vi "PicoScopeospaExampleRapidBlockBulkOverlapped.vi"() -> ()   [LabVIEW 2010]
uses:
  shared/PicoBuffers.ctl
  <vilib>/Waveform/DWDTOps.llb/DWDT Analog to Digital.vi
  PicoScopepsospaLib/PicoScopeospaDigitalChannelSettings.ctl
  PicoScopepsospaLib/PicoScopeospaAnalogChannelSettings.ctl
  shared/Buffer and Transfer Settings.ctl
  shared/Acquisition Settings.ctl
  shared/Segment Range.ctl
panel:
  in  "timeIntervalRequested":dbl=2e-10 format="%#6_6p"
  in  "Write to file":bool
  in  "Channels":T1={"Channel A Settings "={"Enabled"=TRUE, "Coupling"=1, "Range"=8, "Analogue Offset"=0.0, "BandWidth"=0, "PROBE_RANGE_INFO"=0}, "Channel B Settings "={"Enabled"=FALSE, "Coupling"=1, "Range"=8, "Analogue Offset"=0.0, "BandWidth"=0, "PROBE_RANGE_INFO"=0}, "Channel C Settings "={"Enabled"=FALSE, "Coupling"=1, "Range"=8, "Analogue Offset"=0.0, "BandWidth"=0, "PROBE_RANGE_INFO"=0}, "Channel D Settings "={"Enabled"=FALSE, "Coupling"=1, "Range"=8, "Analogue Offset"=0.0, "BandWidth"=0, "PROBE_RANGE_INFO"=0}, "Channel E Settings "={"Enabled"=FALSE, "Coupling"=50, "Range"=5, "Analogue Offset"=0.0, "BandWidth"=0, "PROBE_RANGE_INFO"=0}, "Channel F Settings "={"Enabled"=FALSE, "Coupling"=50, "Range"=5, "Analogue Offset"=0.0, "BandWidth"=0, "PROBE_RANGE_INFO"=0}, "Channel G Settings "={"Enabled"=FALSE, "Coupling"=50, "Range"=5, "Analogue Offset"=0.0, "BandWidth"=0, "PROBE_RANGE_INFO"=0}, "Channel H Settings "={"Enabled"=FALSE, "Coupling"=50, "Range"=5, "Analogue Offset"=0.0, "BandWidth"=0, "PROBE_RANGE_INFO"=0}} {"Channel H Settings"."PROBE_RANGE_INFO" items=["PROBE_NONE_NV"=0, "X1_PROBE_NV"=1, "X10_PROBE_NV"=10]; "Channel H Settings"."BandWidth" items=["Full"=0, "100kHz"=100000, "20kHz"=200000, "1MHz"=1000000, "20MHz"=20000000, "25MHz"=25000000, "50MHz"=50000000, "200MHz"=200000000, "250MHz"=250000000, "500MHz"=500000000]; "Channel H Settings"."Range" items=["10mV"=0, "20mV"=1, "50mV"=2, "100mV"=3, "200mV"=4, "500mV"=5, "1V"=6, "2V"=7, "5V"=8, "10V"=9, "20V"=10, "50V"=11, "100V"=12, "200V"=13, "x10_Probe_100mV"=32, "x10_Probe_200mV"=33, "x10_Probe_500mV"=34, "x10_Probe_1V"=35, "x10_Probe_2V"=36, "x10_Probe_5V"=37, "x10_Probe_10V"=38, "x10_Probe_20V"=39, "x10_Probe_50V"=40, "x10_Probe_100V"=41, "x10_Probe_200V"=42, "x10_Probe_500V"=43, "CURRENT_CLAMP_60A_2A"=10500, "CURRENT_CLAMP_60A_5A"=10501, "CURRENT_CLAMP_60A_10A"=10502, "CURRENT_CLAMP_60A_20A"=10503, "CURRENT_CLAMP_60A_50A"=10504, "CURRENT_CLAMP_60A_60A"=10505, "CURRENT_CLAMP_60A_V2_0_5A"=10600, "CURRENT_CLAMP_60A_V2_1A"=10601, "CURRENT_CLAMP_60A_V2_2A"=10602, "CURRENT_CLAMP_60A_V2_5A"=10603, "CURRENT_CLAMP_60A_V2_10A"=10604, "CURRENT_CLAMP_60A_V2_20A"=10605, "CURRENT_CLAMP_60A_V2_50A"=10606, "CURRENT_CLAMP_60A_V2_60A"=10607, "RESISTANCE_LEAD_NEG5_TO_20OHM"=7000, "RESISTANCE_LEAD_NEG50_TO_200OHM"=7001, "RESISTANCE_LEAD_NEG500_TO_2KOHM"=7002, "RESISTANCE_LEAD_NEG5K_TO_20KOHM"=7003, "RESISTANCE_LEAD_NEG50K_TO_LEAD_200KOHM"=7004, "RESISTANCE_LEAD_NEG500K_TO_LEAD_2MOHM"=7005, "RESISTANCE_LEAD_DIODE_TEST"=7006, "HT_NEG3_TO_5KV"=8950, "HT_NEG3_TO_10KV"=8951, "HT_NEG5_TO_20KV"=8952, "HT_NEG5_TO_50KV"=8953, "HT_NEG5_TO_100KV"=8954, "HT_NEG3_TO_5KV_INVERTED"=8955, "HT_NEG3_TO_10KV_INVERTED"=8956, "HT_NEG5_TO_20KV_INVERTED"=8957, "HT_NEG5_TO_50KV_INVERTED"=8958, "HT_NEG5_TO_100KV_INVERTED"=8959, "TEMPERATURE_NEG50_TO_150DEGC"=9000, "PRESSURE_SENSOR_-100k-150k_PASCALS"=9100, "PRESSURE_SENSOR_-100k_TO_400k_PASCALS"=9101, "PRESSURE_SENSOR_-200k_TO_800k_PASCALS"=9102, "PRESSURE_SENSOR_-400k_TO_1600k_PASCALS"=9103, "PRESSURE_SENSOR_-400k_TO_3400k_PASCALS"=9104, "PRESSURE_SENSOR_-150k_TO_1350k_PASCALS"=9105]; "Channel H Settings"."Coupling" items=["AC"=0, "DC 1M Ohm"=1, "DC 50 Ohm"=50]; "Channel G Settings"."PROBE_RANGE_INFO" items=["PROBE_NONE_NV"=0, "X1_PROBE_NV"=1, "X10_PROBE_NV"=10]; "Channel G Settings"."BandWidth" items=["Full"=0, "100kHz"=100000, "20kHz"=200000, "1MHz"=1000000, "20MHz"=20000000, "25MHz"=25000000, "50MHz"=50000000, "200MHz"=200000000, "250MHz"=250000000, "500MHz"=500000000]; "Channel G Settings"."Range" items=["10mV"=0, "20mV"=1, "50mV"=2, "100mV"=3, "200mV"=4, "500mV"=5, "1V"=6, "2V"=7, "5V"=8, "10V"=9, "20V"=10, "50V"=11, "100V"=12, "200V"=13, "x10_Probe_100mV"=32, "x10_Probe_200mV"=33, "x10_Probe_500mV"=34, "x10_Probe_1V"=35, "x10_Probe_2V"=36, "x10_Probe_5V"=37, "x10_Probe_10V"=38, "x10_Probe_20V"=39, "x10_Probe_50V"=40, "x10_Probe_100V"=41, "x10_Probe_200V"=42, "x10_Probe_500V"=43, "CURRENT_CLAMP_60A_2A"=10500, "CURRENT_CLAMP_60A_5A"=10501, "CURRENT_CLAMP_60A_10A"=10502, "CURRENT_CLAMP_60A_20A"=10503, "CURRENT_CLAMP_60A_50A"=10504, "CURRENT_CLAMP_60A_60A"=10505, "CURRENT_CLAMP_60A_V2_0_5A"=10600, "CURRENT_CLAMP_60A_V2_1A"=10601, "CURRENT_CLAMP_60A_V2_2A"=10602, "CURRENT_CLAMP_60A_V2_5A"=10603, "CURRENT_CLAMP_60A_V2_10A"=10604, "CURRENT_CLAMP_60A_V2_20A"=10605, "CURRENT_CLAMP_60A_V2_50A"=10606, "CURRENT_CLAMP_60A_V2_60A"=10607, "RESISTANCE_LEAD_NEG5_TO_20OHM"=7000, "RESISTANCE_LEAD_NEG50_TO_200OHM"=7001, "RESISTANCE_LEAD_NEG500_TO_2KOHM"=7002, "RESISTANCE_LEAD_NEG5K_TO_20KOHM"=7003, "RESISTANCE_LEAD_NEG50K_TO_LEAD_200KOHM"=7004, "RESISTANCE_LEAD_NEG500K_TO_LEAD_2MOHM"=7005, "RESISTANCE_LEAD_DIODE_TEST"=7006, "HT_NEG3_TO_5KV"=8950, "HT_NEG3_TO_10KV"=8951, "HT_NEG5_TO_20KV"=8952, "HT_NEG5_TO_50KV"=8953, "HT_NEG5_TO_100KV"=8954, "HT_NEG3_TO_5KV_INVERTED"=8955, "HT_NEG3_TO_10KV_INVERTED"=8956, "HT_NEG5_TO_20KV_INVERTED"=8957, "HT_NEG5_TO_50KV_INVERTED"=8958, "HT_NEG5_TO_100KV_INVERTED"=8959, "TEMPERATURE_NEG50_TO_150DEGC"=9000, "PRESSURE_SENSOR_-100k-150k_PASCALS"=9100, "PRESSURE_SENSOR_-100k_TO_400k_PASCALS"=9101, "PRESSURE_SENSOR_-200k_TO_800k_PASCALS"=9102, "PRESSURE_SENSOR_-400k_TO_1600k_PASCALS"=9103, "PRESSURE_SENSOR_-400k_TO_3400k_PASCALS"=9104, "PRESSURE_SENSOR_-150k_TO_1350k_PASCALS"=9105]; "Channel G Settings"."Coupling" items=["AC"=0, "DC 1M Ohm"=1, "DC 50 Ohm"=50]; "Channel F Settings"."PROBE_RANGE_INFO" items=["PROBE_NONE_NV"=0, "X1_PROBE_NV"=1, "X10_PROBE_NV"=10]; "Channel F Settings"."BandWidth" items=["Full"=0, "100kHz"=100000, "20kHz"=200000, "1MHz"=1000000, "20MHz"=20000000, "25MHz"=25000000, "50MHz"=50000000, "200MHz"=200000000, "250MHz"=250000000, "500MHz"=500000000]; "Channel F Settings"."Range" items=["10mV"=0, "20mV"=1, "50mV"=2, "100mV"=3, "200mV"=4, "500mV"=5, "1V"=6, "2V"=7, "5V"=8, "10V"=9, "20V"=10, "50V"=11, "100V"=12, "200V"=13, "x10_Probe_100mV"=32, "x10_Probe_200mV"=33, "x10_Probe_500mV"=34, "x10_Probe_1V"=35, "x10_Probe_2V"=36, "x10_Probe_5V"=37, "x10_Probe_10V"=38, "x10_Probe_20V"=39, "x10_Probe_50V"=40, "x10_Probe_100V"=41, "x10_Probe_200V"=42, "x10_Probe_500V"=43, "CURRENT_CLAMP_60A_2A"=10500, "CURRENT_CLAMP_60A_5A"=10501, "CURRENT_CLAMP_60A_10A"=10502, "CURRENT_CLAMP_60A_20A"=10503, "CURRENT_CLAMP_60A_50A"=10504, "CURRENT_CLAMP_60A_60A"=10505, "CURRENT_CLAMP_60A_V2_0_5A"=10600, "CURRENT_CLAMP_60A_V2_1A"=10601, "CURRENT_CLAMP_60A_V2_2A"=10602, "CURRENT_CLAMP_60A_V2_5A"=10603, "CURRENT_CLAMP_60A_V2_10A"=10604, "CURRENT_CLAMP_60A_V2_20A"=10605, "CURRENT_CLAMP_60A_V2_50A"=10606, "CURRENT_CLAMP_60A_V2_60A"=10607, "RESISTANCE_LEAD_NEG5_TO_20OHM"=7000, "RESISTANCE_LEAD_NEG50_TO_200OHM"=7001, "RESISTANCE_LEAD_NEG500_TO_2KOHM"=7002, "RESISTANCE_LEAD_NEG5K_TO_20KOHM"=7003, "RESISTANCE_LEAD_NEG50K_TO_LEAD_200KOHM"=7004, "RESISTANCE_LEAD_NEG500K_TO_LEAD_2MOHM"=7005, "RESISTANCE_LEAD_DIODE_TEST"=7006, "HT_NEG3_TO_5KV"=8950, "HT_NEG3_TO_10KV"=8951, "HT_NEG5_TO_20KV"=8952, "HT_NEG5_TO_50KV"=8953, "HT_NEG5_TO_100KV"=8954, "HT_NEG3_TO_5KV_INVERTED"=8955, "HT_NEG3_TO_10KV_INVERTED"=8956, "HT_NEG5_TO_20KV_INVERTED"=8957, "HT_NEG5_TO_50KV_INVERTED"=8958, "HT_NEG5_TO_100KV_INVERTED"=8959, "TEMPERATURE_NEG50_TO_150DEGC"=9000, "PRESSURE_SENSOR_-100k-150k_PASCALS"=9100, "PRESSURE_SENSOR_-100k_TO_400k_PASCALS"=9101, "PRESSURE_SENSOR_-200k_TO_800k_PASCALS"=9102, "PRESSURE_SENSOR_-400k_TO_1600k_PASCALS"=9103, "PRESSURE_SENSOR_-400k_TO_3400k_PASCALS"=9104, "PRESSURE_SENSOR_-150k_TO_1350k_PASCALS"=9105]; "Channel F Settings"."Coupling" items=["AC"=0, "DC 1M Ohm"=1, "DC 50 Ohm"=50]; "Channel E Settings"."PROBE_RANGE_INFO" items=["PROBE_NONE_NV"=0, "X1_PROBE_NV"=1, "X10_PROBE_NV"=10]; "Channel E Settings"."BandWidth" items=["Full"=0, "100kHz"=100000, "20kHz"=200000, "1MHz"=1000000, "20MHz"=20000000, "25MHz"=25000000, "50MHz"=50000000, "200MHz"=200000000, "250MHz"=250000000, "500MHz"=500000000]; "Channel E Settings"."Range" items=["10mV"=0, "20mV"=1, "50mV"=2, "100mV"=3, "200mV"=4, "500mV"=5, "1V"=6, "2V"=7, "5V"=8, "10V"=9, "20V"=10, "50V"=11, "100V"=12, "200V"=13, "x10_Probe_100mV"=32, "x10_Probe_200mV"=33, "x10_Probe_500mV"=34, "x10_Probe_1V"=35, "x10_Probe_2V"=36, "x10_Probe_5V"=37, "x10_Probe_10V"=38, "x10_Probe_20V"=39, "x10_Probe_50V"=40, "x10_Probe_100V"=41, "x10_Probe_200V"=42, "x10_Probe_500V"=43, "CURRENT_CLAMP_60A_2A"=10500, "CURRENT_CLAMP_60A_5A"=10501, "CURRENT_CLAMP_60A_10A"=10502, "CURRENT_CLAMP_60A_20A"=10503, "CURRENT_CLAMP_60A_50A"=10504, "CURRENT_CLAMP_60A_60A"=10505, "CURRENT_CLAMP_60A_V2_0_5A"=10600, "CURRENT_CLAMP_60A_V2_1A"=10601, "CURRENT_CLAMP_60A_V2_2A"=10602, "CURRENT_CLAMP_60A_V2_5A"=10603, "CURRENT_CLAMP_60A_V2_10A"=10604, "CURRENT_CLAMP_60A_V2_20A"=10605, "CURRENT_CLAMP_60A_V2_50A"=10606, "CURRENT_CLAMP_60A_V2_60A"=10607, "RESISTANCE_LEAD_NEG5_TO_20OHM"=7000, "RESISTANCE_LEAD_NEG50_TO_200OHM"=7001, "RESISTANCE_LEAD_NEG500_TO_2KOHM"=7002, "RESISTANCE_LEAD_NEG5K_TO_20KOHM"=7003, "RESISTANCE_LEAD_NEG50K_TO_LEAD_200KOHM"=7004, "RESISTANCE_LEAD_NEG500K_TO_LEAD_2MOHM"=7005, "RESISTANCE_LEAD_DIODE_TEST"=7006, "HT_NEG3_TO_5KV"=8950, "HT_NEG3_TO_10KV"=8951, "HT_NEG5_TO_20KV"=8952, "HT_NEG5_TO_50KV"=8953, "HT_NEG5_TO_100KV"=8954, "HT_NEG3_TO_5KV_INVERTED"=8955, "HT_NEG3_TO_10KV_INVERTED"=8956, "HT_NEG5_TO_20KV_INVERTED"=8957, "HT_NEG5_TO_50KV_INVERTED"=8958, "HT_NEG5_TO_100KV_INVERTED"=8959, "TEMPERATURE_NEG50_TO_150DEGC"=9000, "PRESSURE_SENSOR_-100k-150k_PASCALS"=9100, "PRESSURE_SENSOR_-100k_TO_400k_PASCALS"=9101, "PRESSURE_SENSOR_-200k_TO_800k_PASCALS"=9102, "PRESSURE_SENSOR_-400k_TO_1600k_PASCALS"=9103, "PRESSURE_SENSOR_-400k_TO_3400k_PASCALS"=9104, "PRESSURE_SENSOR_-150k_TO_1350k_PASCALS"=9105]; "Channel E Settings"."Coupling" items=["AC"=0, "DC 1M Ohm"=1, "DC 50 Ohm"=50]; "Channel D Settings"."BandWidth" items=["Full"=0, "100kHz"=100000, "20kHz"=200000, "1MHz"=1000000, "20MHz"=20000000, "25MHz"=25000000, "50MHz"=50000000, "100MHz"=100000000, "200MHz"=200000000, "250MHz"=250000000, "350MHz"=350000000, "500MHz"=500000000]; "Channel D Settings"."PROBE_RANGE_INFO" items=["PROBE_NONE_NV"=0, "X1_PROBE_NV"=1, "X10_PROBE_NV"=10]; "Channel D Settings"."Range" items=["10mV", "20mV", "50mV", "100mV", "200mV", "500mV", "1V", "2V", "5V", "10V", "20V", "50V", "100V", "200V"]; "Channel D Settings"."Coupling" items=["AC"=0, "DC 1M Ohm"=1, "DC 50 Ohm"=50]; "Channel C Settings"."BandWidth" items=["Full"=0, "100kHz"=100000, "20kHz"=200000, "1MHz"=1000000, "20MHz"=20000000, "25MHz"=25000000, "50MHz"=50000000, "100MHz"=100000000, "200MHz"=200000000, "250MHz"=250000000, "350MHz"=350000000, "500MHz"=500000000]; "Channel C Settings"."PROBE_RANGE_INFO" items=["PROBE_NONE_NV"=0, "X1_PROBE_NV"=1, "X10_PROBE_NV"=10]; "Channel C Settings"."Range" items=["10mV", "20mV", "50mV", "100mV", "200mV", "500mV", "1V", "2V", "5V", "10V", "20V", "50V", "100V", "200V"]; "Channel C Settings"."Coupling" items=["AC"=0, "DC 1M Ohm"=1, "DC 50 Ohm"=50]; "Channel B Settings"."BandWidth" items=["Full"=0, "100kHz"=100000, "20kHz"=200000, "1MHz"=1000000, "20MHz"=20000000, "25MHz"=25000000, "50MHz"=50000000, "100MHz"=100000000, "200MHz"=200000000, "250MHz"=250000000, "350MHz"=350000000, "500MHz"=500000000]; "Channel B Settings"."PROBE_RANGE_INFO" items=["PROBE_NONE_NV"=0, "X1_PROBE_NV"=1, "X10_PROBE_NV"=10]; "Channel B Settings"."Range" items=["10mV", "20mV", "50mV", "100mV", "200mV", "500mV", "1V", "2V", "5V", "10V", "20V", "50V", "100V", "200V"]; "Channel B Settings"."Coupling" items=["AC"=0, "DC 1M Ohm"=1, "DC 50 Ohm"=50]; "Channel A Settings"."PROBE_RANGE_INFO" items=["PROBE_NONE_NV"=0, "X1_PROBE_NV"=1, "X10_PROBE_NV"=10]; "Channel A Settings"."Range" items=["10mV", "20mV", "50mV", "100mV", "200mV", "500mV", "1V", "2V", "5V", "10V", "20V", "50V", "100V", "200V"]; "Channel A Settings"."BandWidth" items=["Full"=0, "100kHz"=100000, "20kHz"=200000, "1MHz"=1000000, "20MHz"=20000000, "25MHz"=25000000, "50MHz"=50000000, "100MHz"=100000000, "200MHz"=200000000, "250MHz"=250000000, "350MHz"=350000000, "500MHz"=500000000]; "Channel A Settings"."Coupling" items=["AC"=0, "DC 1M Ohm"=1, "DC 50 Ohm"=50]}
  out "overflow":i16[](array[numeric])=[1023] format="%010d"
  out "Trigger Offsets":cluster{"Samples":u64, "Time (seconds)":dbl}[](array[cluster]) {"Time (seconds)" format="%#_5p"}
  in  "Stop Display":bool
  out "Capture Complete":bool
  in  "Run":bool
  in  "Display Buffer Index":i32
  in  "Segment Range":T2={"fromSegmentIndex"=0, "toSegmentIndex"=9} {"toSegmentIndex" format="%.4p"; "fromSegmentIndex" format="%.4p"}
  in  "nSegments":u64=10 format="%.4p"
  out "error out":errorcluster
  in  "Data file":path=path "PicoScopeospaExampleRapidBlock ChA Data"
  in  "Digital Channels":T3={"Port 0 Settings "={"Enabled"=FALSE, "Threshold Level (Volts)"=3.0}, "Port 1 Settings"={"Enabled"=FALSE, "Threshold Level (Volts)"=3.0}} {"Port 1 Settings"."Threshold Level (Volts)" format="%#_4p"; "Port 0 Settings"."Threshold Level (Volts)" format="%#_4p"}
  in  "Trigger Settings":T4={"Trigger Enabled"=FALSE, "Trigger Threshold (Volts)"=0.0, "Trigger Direction"=2, "Trigger Delay (samples)"=0, "Auto Trigger Time (us)"=1000000, "Trigger Source"=0} {"Trigger Source" items=["Channel A"=0, "Channel B"=1, "Channel C"=2, "Channel D"=3, "Channel E"=4, "Channel F"=5, "Channel G"=6, "Channel H"=7, "Port 0"=128, "Port 1"=129, "Trigger AUX"=1001]; "Auto Trigger Time (us)" format="%.4p"; "Trigger Direction" items=["Above", "Below", "Rising", "Falling", "Rising or Falling"]; "Trigger Threshold (Volts)" format="%#_6p"}
  in  "Buffer and Transfer Settings":T5={"startIndex"=0, "Samples"=10000000, "Down Sample Ratio"=10, "Down-Sample Mode"=2147483648} {"Down-Sample Mode" items=["RAW none"=2147483648, "None"=0, "Aggregate"=1, "Decimate"=2, "Average"=4]; "Down Sample Ratio" step=1; "Samples" format="%_6p"}
  in  "Acquisition Settings":T6={"preTriggerSamples"=0, "postTriggerSamples"=10000000, "timebase"=5} {"postTriggerSamples" format="%_6p"; "preTriggerSamples" format="%_6p"}
  out "Properties Panel":T7 {"Max Total Capture Time Available (sec)" format="%.3p"; "Sample Frequency" format="%.6p"; "Sample Rate" format="%.3p"; "Max Samples Available" format="%_6p"; "Total Capture Time (sec)" format="%.3p"}
  out "Port 0":digitalwaveform(graph)={"t0"=timestamp(0 s since 1904-01-01), "dt"=8e-09, "Y"={"transitions"=[], "data"=[]}}
  in  "stop":bool
  out "Analog Channels":cluster{i32, dbl, "Data":dbl[]}[](graph)
  out "Device Info":T8={"PICO_DRIVER_VERSION"="", "PICO_USB_VERSION"="", "PICO_HARDWARE_VERSION"="", "PICO_VARIANT_INFO"="", "PICO_BATCH_AND_SERIAL"="", "PICO_CAL_DATE"="", "PICO_KERNEL_VERSION"="", "PICO_DIGITAL_HARDWARE_VERSION"="", "PICO_ANALOGUE_HARDWARE_VERSION"="", "PICO_FIRMWARE_VERSION_1"="", "PICO_FIRMWARE_VERSION_2"="", "PICO_IPP_VERSION"="", "PICO_DRIVER_PATH"="", "PICO_FIRMWARE_VERSION_3"="", "PICO_FRONT_PANEL_FIRMWARE_VERSION"="", "Number of Channels"=8, "MSO"=FALSE}
  out "Pico ospa Units":string
  in  "Resolution":u32(ring)=10 items=["8-bit"=0, "12-bit"=1, "14-bit"=2, "15-bit"=3, "16-bit"=4, "10-bit"=10]
  in  "Serial Number":string
  in  "Use Serial Number":bool
  in  "error in (no error)":errorcluster
  # "Bit 0 = ChA"
  # "D8-D15"
  # "DO-D7"
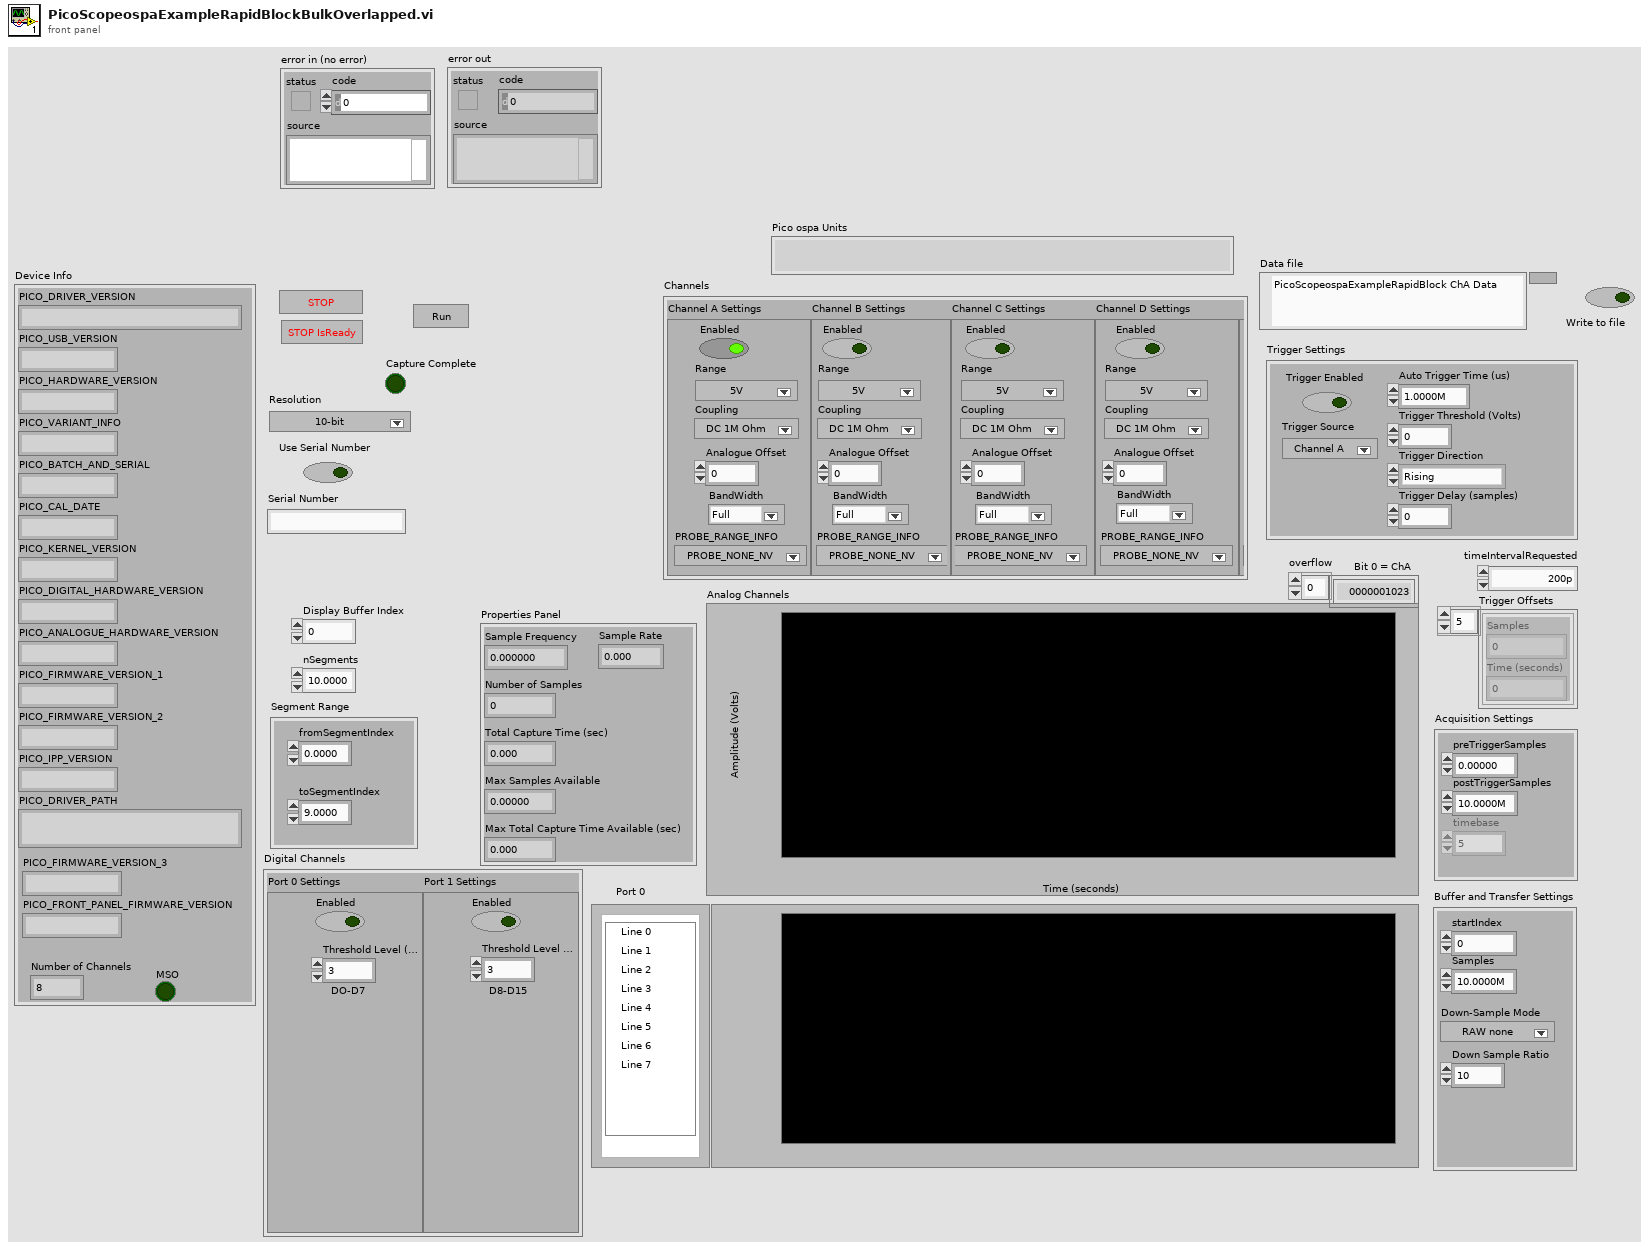
[diagram p1: front panel]
types:
  T1 = typedef "PicoScopeospaAnalogChannelSettings.ctl" = cluster{"Channel A Settings ":cluster{"Enabled":bool, "Coupling":i16, "Range":u16, "Analogue Offset":dbl, "BandWidth":u32, "PROBE_RANGE_INFO":u32}, "Channel B Settings ":cluster{"Enabled":bool, "Coupling":i16, "Range":u16, "Analogue Offset":dbl, "BandWidth":u32, "PROBE_RANGE_INFO":u32}, "Channel C Settings ":cluster{"Enabled":bool, "Coupling":i16, "Range":u16, "Analogue Offset":dbl, "BandWidth":u32, "PROBE_RANGE_INFO":u32}, "Channel D Settings ":cluster{"Enabled":bool, "Coupling":i16, "Range":u16, "Analogue Offset":dbl, "BandWidth":u32, "PROBE_RANGE_INFO":u32}, "Channel E Settings ":cluster{"Enabled":bool, "Coupling":i16, "Range":u16, "Analogue Offset":dbl, "BandWidth":u32, "PROBE_RANGE_INFO":u32}, "Channel F Settings ":cluster{"Enabled":bool, "Coupling":i16, "Range":u16, "Analogue Offset":dbl, "BandWidth":u32, "PROBE_RANGE_INFO":u32}, "Channel G Settings ":cluster{"Enabled":bool, "Coupling":i16, "Range":u16, "Analogue Offset":dbl, "BandWidth":u32, "PROBE_RANGE_INFO":u32}, "Channel H Settings ":cluster{"Enabled":bool, "Coupling":i16, "Range":u16, "Analogue Offset":dbl, "BandWidth":u32, "PROBE_RANGE_INFO":u32}}
  T2 = typedef "Segment Range.ctl" = cluster{"fromSegmentIndex":u64, "toSegmentIndex":u64}
  T3 = typedef "PicoScopeospaDigitalChannelSettings.ctl" = cluster{"Port 0 Settings ":cluster{"Enabled":bool, "Threshold Level (Volts)":dbl}, "Port 1 Settings":cluster{"Enabled":bool, "Threshold Level (Volts)":dbl}}
  T4 = cluster{"Trigger Enabled":bool, "Trigger Threshold (Volts)":dbl, "Trigger Direction":u16, "Trigger Delay (samples)":u64, "Auto Trigger Time (us)":u32, "Trigger Source":u32}
  T5 = typedef "Buffer and Transfer Settings.ctl" = cluster{"startIndex":u64, "Samples":u64, "Down Sample Ratio":u64, "Down-Sample Mode":u32}
  T6 = typedef "Acquisition Settings.ctl" = cluster{"preTriggerSamples":u64, "postTriggerSamples":u64, "timebase":u32}
  T7 = cluster{"Sample Frequency":dbl, "Sample Rate":dbl, "Max Samples Available":u64, "Number of Samples":u64, "Total Capture Time (sec) ":dbl, "Max Total Capture Time Available (sec)":dbl}
  T8 = cluster{"PICO_DRIVER_VERSION":string, "PICO_USB_VERSION":string, "PICO_HARDWARE_VERSION":string, "PICO_VARIANT_INFO":string, "PICO_BATCH_AND_SERIAL":string, "PICO_CAL_DATE":string, "PICO_KERNEL_VERSION":string, "PICO_DIGITAL_HARDWARE_VERSION":string, "PICO_ANALOGUE_HARDWARE_VERSION":string, "PICO_FIRMWARE_VERSION_1":string, "PICO_FIRMWARE_VERSION_2":string, "PICO_IPP_VERSION":string, "PICO_DRIVER_PATH":string, "PICO_FIRMWARE_VERSION_3":string, "PICO_FRONT_PANEL_FIRMWARE_VERSION":string, "Number of Channels":i16, "MSO":bool}
  T9 = typedef "PicoBuffers.ctl" = cluster{"Max Buffer Pointers":u64[][][], "Min Buffer Pointers":u64[][][], "StreamingDataInfo":cluster{"Channel":u32, "Down-Sample Mode":u32, "PICO_DATA_TYPE":enum32{"PICO_INT8_T", "PICO_INT16_T", "PICO_INT32_T", "PICO_UINT32_T", "PICO_INT64_T", ""}, "Samples":i32, "bufferIndex":u64, "startIndex":i32, "overflow":i16}[][]}
  T10 = enum16{"open", "open or create", "create or replace", "create", "open (read-only)"}
  T11 = cluster{"Channel A Buffer":i16[], "Channel B Buffer":i16[], "Channel C Buffer":i16[], "Channel D Buffer":i16[], "Channel E Buffer":i16[], "Channel F Buffer":i16[], "Channel G Buffer":i16[], "Channel H Buffer":i16[], "Port 0 Buffer":i16[], "Port 1 Buffer":i16[]}[]
  T12 = cluster{"Channel A Buffer":i16[], "Channel B Buffer":i16[], "Channel C Buffer":i16[], "Channel D Buffer":i16[], "Channel E Buffer":i16[], "Channel F Buffer":i16[], "Channel G Buffer":i16[], "Channel H Buffer":i16[], "Port 0 Buffer":i16[], "Port 1 Buffer":i16[]}
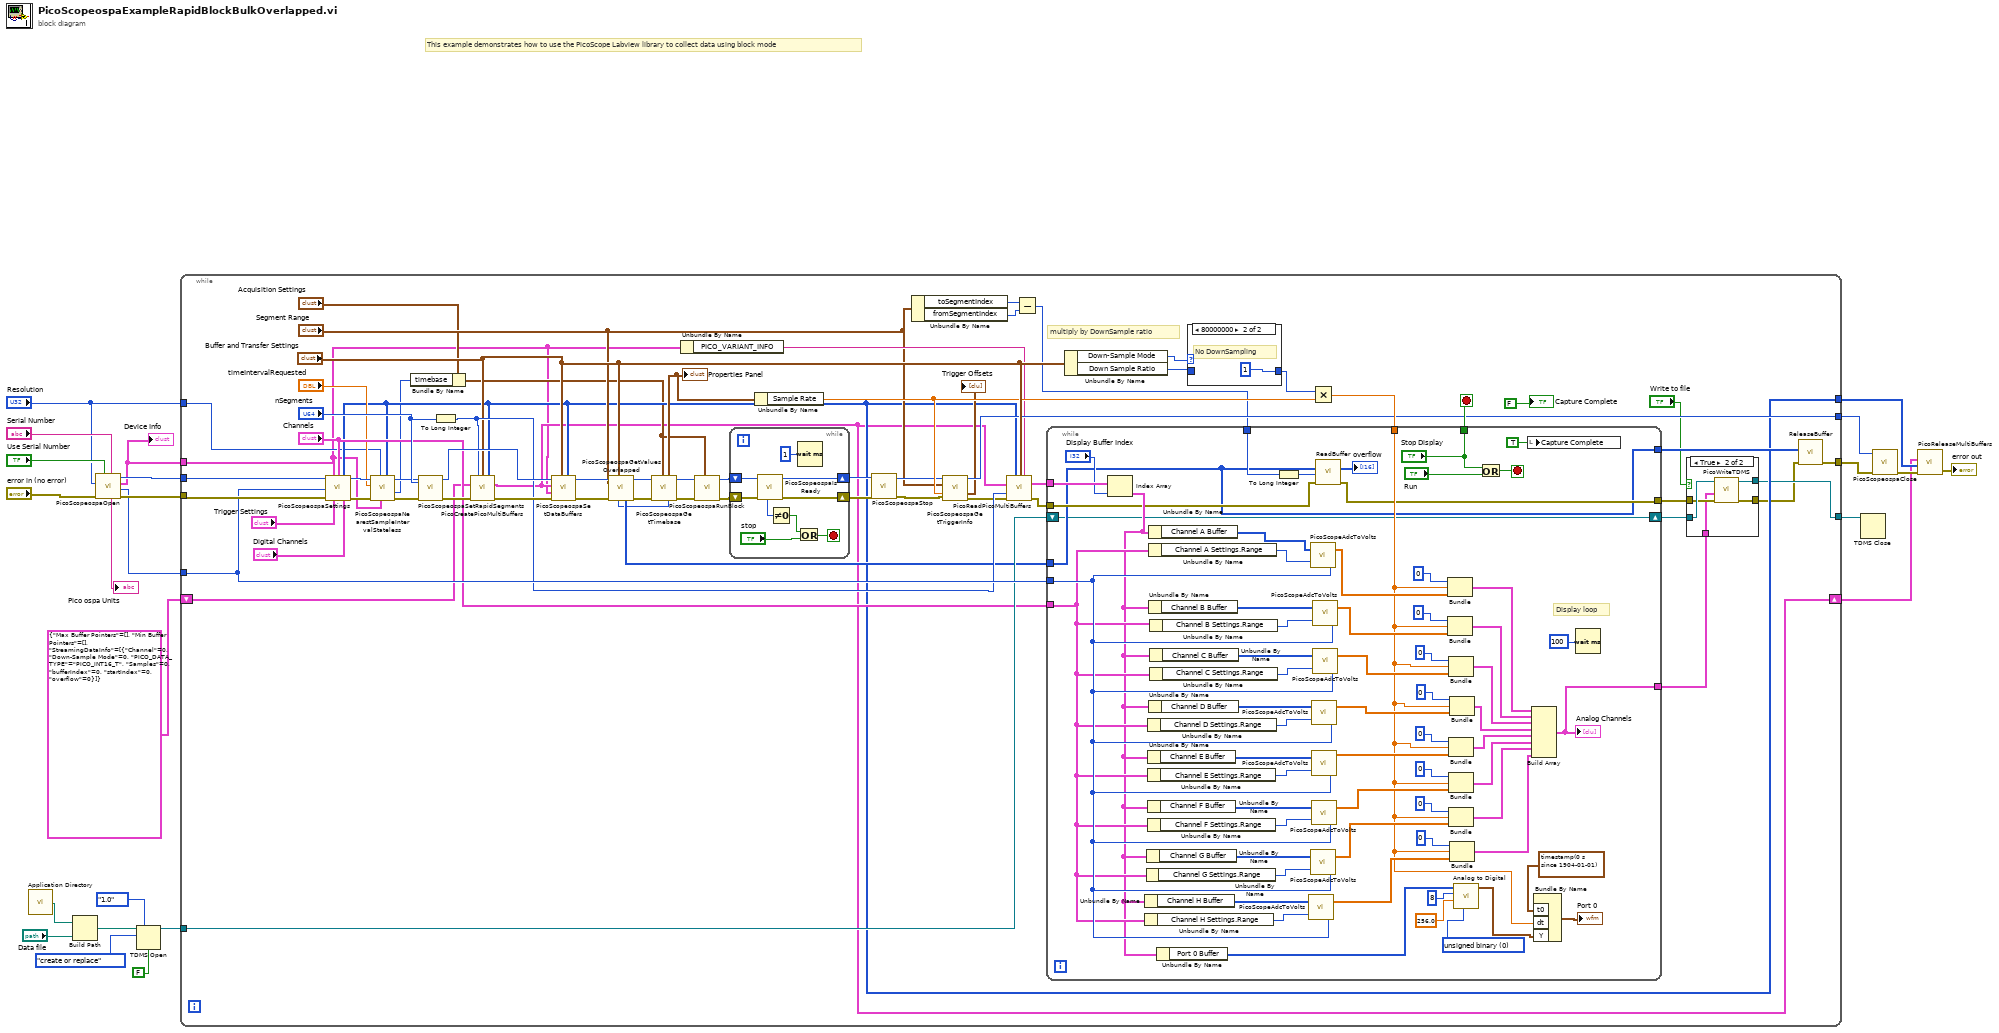
[diagram p0: block diagram]
diagram:
  # "This example demonstrates how to use the PicoScope Labview library to collect data using block mode"
  n1 = call <vilib>:"Application Directory.vi"() -> ("Application Directory"=w7:path)
  n2 = Build Path(base path=w7, name or relative path="Data file") -> (appended path=w8:path)
  n3 = call "PicoScopeospaOpen.vi"("Serial Number"="Serial Number", "Use Serial Number"="Use Serial Number", "error in (no error)"="error in (no error)", "Resolution"="Resolution") -> ("error out"=w20:errorcluster, "Max ADC value"=w18:i16, "Device Info"=w17:T8, "handle out"=w21:i16, "psospa Units"=→"Pico ospa Units":string)  [unwired: 2 in, 1 out]
  "Device Info" <- w17
  n4 = TDMS Open(6:FALSE ("disable buffering? (T)"), 7:enum16{"1.0", "2.0"}."1.0" ("file format version (2.0)"), 10:T10."create or replace" ("operation (0:open)"), 11:w8) -> (3:w5:refnum<k34>)  [unwired: 2 in, 1 out]
  n5 = while {
    tunnel: w17 -> [w25]
    tunnel: w18 -> [w88]
    tunnel: w21 -> [w90]
    tunnel: [w60] -> w14
    tunnel: w20 -> [w89]
    tunnel: [w45] -> w15
    tunnel: [w38] -> w16
    tunnel: [w29] -> w6
    tunnel: w5 -> [w84]
    tunnel: "Resolution" -> [w37]
    shift-right: [w26] -> w1
    shift-left: T9 {"Max Buffer Pointers"=[], "Min Buffer Pointers"=[], "StreamingDataInfo"=[[{"Channel"=0, "Down-Sample Mode"=0, "PICO_DATA_TYPE"=enum."PICO_INT16_T", "Samples"=0, "bufferIndex"=0, "startIndex"=0, "overflow"=0}]]} ("Data Pointers") -> [w27]
    stop <- w66 stop-if-true
    # "multiply by DownSample ratio"
    n6 = call "PicoScopeospaSettings.vi"("handle in"=w90, "Device Info"=w25, "Channels"="Channels", "Max ADC value"=w88, "error in (no error)"=w89, "Trigger Settings"="Trigger Settings", "Digital Channels"="Digital Channels") -> ("Enabled array"=w38:i16[], "handle out"=w40:i16, "error out"=w43:errorcluster)  [unwired: 6 in]
    n7 = call "PicoScopeospaNearestSampleIntervalStateless.vi"("Enabled array"=w38, "Device Info"=w25, "Resolution"=w37, "error in (no error)"=w43, "timeIntervalRequested"="timeIntervalRequested", "handle in"=w40) -> ("error out"=w42:errorcluster, "timebase"=w36:u32, "handle out"=w41:i16)  [unwired: 2 in, 1 out]
    n8 = Bundle By Name(cluster="Acquisition Settings", "timebase"=w36) -> (w34:T6)
    n9 = call "PicoScopeospaSetRapidSegments.vi"("nSegments"="nSegments", "error in (no error)"=w42, "handle in"=w41) -> ("error out"=w83:errorcluster, "handle out"=w82:i16)  [unwired: 6 in, 1 out]
    n10 = To Long Integer(number="nSegments") -> (32bit integer=w78:i32)
    n11 = call "PicoCreatePicoMultiBuffers.vi"("Number of Buffers"=w78, "Buffer and Transfer Settings"="Buffer and Transfer Settings", "enabled array"=w38, "Data Pointers In"=w27, "error in (no error)"=w83) -> ("Data Pointers"=w26:T9, "error out"=w85:errorcluster)  [unwired: 9 in]
    n12 = call "PicoScopeospaSetDataBuffers.vi"("enabled array"=w38, "Buffer and Transfer Settings"="Buffer and Transfer Settings", "error in (no error)"=w85, "Device Info"=w25, "Data Pointers In"=w26, "handle in"=w82) -> ("error out"=w81:errorcluster, "handle out"=w80:i16)  [unwired: 4 in]
    n13 = call "PicoScopeospaGetValuesOverlapped.vi"("Segment Range"="Segment Range", "Buffer and Transfer Settings"="Buffer and Transfer Settings", "error in (no error)"=w81, "handle in"=w80) -> ("error out"=w63:errorcluster, "handle out"=w62:i16, "Pointer to Overflow"=w52:u64[], "noOfSamples"=w44:u64)  [unwired: 4 in]
    n14 = call "PicoScopeospaGetTimebase.vi"("Number of Samples"=w44, "Acquisition Settings"=w34, "error in (no error)"=w63, "handle in"=w62) -> ("error out"=w70:errorcluster, "handle out"=w71:i16, "Properties Panel"=w74:T7)  [unwired: 5 in]
    "Properties Panel" <- w74
    n15 = Unbundle By Name(w25) -> ("PICO_VARIANT_INFO"=w53:string)
    n16 = call "PicoScopeospaRunBlock.vi"("Acquisition Settings"=w34, "error in (no error)"=w70, "handle in"=w71) -> ("error out"=w69:errorcluster, "handle out"=w68:i16)  [unwired: 5 in, 2 out]
    n17 = while {
      shift-right: [w171] -> w57
      shift-left: w69 -> [w172]
      shift-right: [w170] -> w54
      shift-left: w68 -> [w169]
      stop <- w167 stop-if-true
      n18 = call "PicoScopeospaIsReady.vi"("error in (no error)"=w172, "handle in"=w169) -> ("error out"=w171:errorcluster, "handle out"=w170:i16, "ready"=w168:i16)  [unwired: 7 in]
      n19 = Not Equal To 0?(x=w168) -> (x != 0?=w166:bool)
      n20 = Or(x=w166, y="stop") -> (x .or. y?=w167:bool)
      n21 = Wait (ms)(milliseconds to wait=u32 1) -> ()  [unwired: 1 out]
    }
    n22 = Unbundle By Name(w74) -> ("Sample Rate"=w59:dbl)
    n23 = call "PicoScopeospaStop.vi"("error in (no error)"=w57, "handle in"=w54) -> ("error out"=w56:errorcluster, "handle out"=w55:i16)  [unwired: 8 in]
    n24 = Unbundle By Name("Segment Range") -> ("toSegmentIndex"=w48:u64, "fromSegmentIndex"=w47:u64)
    n25 = call "PicoScopeospaGetTriggerInfo.vi"("handle in"=w55, "Segment Range"="Segment Range", "Sample Rate"=w59, "error in"=w56) -> ("handle out"=w60:i16, "Trigger Offsets"=→"Trigger Offsets":cluster{"Samples":u64, "Time (seconds)":dbl}[], "error out"=w61:errorcluster)  [unwired: 8 in, 1 out]
    n26 = call "PicoReadPicoMultiBuffers.vi"("enabled array"=w38, "Buffer and Transfer Settings"="Buffer and Transfer Settings", "Variant"=w53, "Data Pointers"=w26, "No of Buffers"=w78, "error in (no error)"=w61) -> ("MultiBuffers (Max or non-aggregated)"=w77:T11, "error out"=w67:errorcluster)  [unwired: 7 in, 1 out]
    n27 = Subtract(x=w48, y=w47) -> (x-y=w49:u64)
    n28 = Unbundle By Name("Buffer and Transfer Settings") -> ("Down-Sample Mode"=w75:u32, "Down Sample Ratio"=w76:u64)
    n29 = case shown="80000000" w75 {
      tunnel: [w173 u64 1 ("Down Sample Ratio")] -> w72
      tunnel: w76 -> [w173 _]
      frame Default {
      }
      frame -2147483648 {
        # "No DownSampling"
      }
    }
    n30 = Multiply(x=w72, y=w59) -> (x*y=w73:dbl)
    n31 = while {
      tunnel: w88 -> [w163]
      tunnel: "Channels" -> [w162]
      tunnel: w77 -> [w115]
      tunnel: w73 -> [w114]
      shift-right: [w99] -> w33
      shift-left: w84 -> [w99]
      tunnel: [w104] -> w32
      tunnel: w67 -> [w105]
      tunnel: ["Stop Display"] -> w66
      tunnel: w52 -> [w100]
      tunnel: w49 -> [w101]
      tunnel: [w100] -> w46
      tunnel: [w98] -> w30
      stop <- w108 stop-if-true
      w123 = u16 0 items=["unsigned binary", "offset binary", "2's complement"] ("data format (offset binary)")
      # "Display loop"
      n32 = Index Array(array=w115, index="Display Buffer Index") -> (element=w113:T12)
      n33 = Unbundle By Name(w113) -> ("Channel H Buffer"=w121:i16[])
      n34 = Unbundle By Name(w162) -> ("Channel H Settings.Range"=w143:u16)
      n35 = Unbundle By Name(w162) -> ("Channel G Settings.Range"=w144:u16)
      n36 = Unbundle By Name(w113) -> ("Channel G Buffer"=w145:i16[])
      n37 = Unbundle By Name(w162) -> ("Channel D Settings.Range"=w150:u16)
      n38 = Unbundle By Name(w113) -> ("Channel E Buffer"=w149:i16[])
      n39 = Unbundle By Name(w162) -> ("Channel E Settings.Range"=w148:u16)
      n40 = Unbundle By Name(w113) -> ("Channel F Buffer"=w147:i16[])
      n41 = Unbundle By Name(w162) -> ("Channel F Settings.Range"=w146:u16)
      n42 = Unbundle By Name(w113) -> ("Channel A Buffer"=w112:i16[])
      n43 = Unbundle By Name(w162) -> ("Channel A Settings.Range"=w160:u16)
      n44 = Unbundle By Name(w113) -> ("Channel B Buffer"=w158:i16[])
      n45 = Unbundle By Name(w113) -> ("Channel D Buffer"=w151:i16[])
      n46 = Unbundle By Name(w162) -> ("Channel B Settings.Range"=w157:u16)
      n47 = Unbundle By Name(w113) -> ("Channel C Buffer"=w153:i16[])
      n48 = Unbundle By Name(w162) -> ("Channel C Settings.Range"=w152:u16)
      n49 = Unbundle By Name(w113) -> ("Port 0 Buffer"=w120:i16[])
      n50 = To Long Integer(number=w101) -> (32bit integer=w102:i32)
      n51 = call "PicoScopeAdcToVolts.vi"("Max_adc"=w163, "Range Index"=w143, "Data"=w121) -> ("Data"=w138:dbl[])
      n52 = call "PicoScopeAdcToVolts.vi"("Max_adc"=w163, "Range Index"=w160, "Data"=w112) -> ("Data"=w116:dbl[])
      n53 = call "PicoScopeAdcToVolts.vi"("Max_adc"=w163, "Range Index"=w144, "Data"=w145) -> ("Data"=w132:dbl[])
      n54 = call "PicoScopeAdcToVolts.vi"("Max_adc"=w163, "Range Index"=w148, "Data"=w149) -> ("Data"=w135:dbl[])
      n55 = call "PicoScopeAdcToVolts.vi"("Max_adc"=w163, "Range Index"=w146, "Data"=w147) -> ("Data"=w131:dbl[])
      n56 = call "PicoScopeAdcToVolts.vi"("Max_adc"=w163, "Range Index"=w150, "Data"=w151) -> ("Data"=w136:dbl[])
      n57 = call "PicoScopeAdcToVolts.vi"("Max_adc"=w163, "Range Index"=w157, "Data"=w158) -> ("Data"=w156:dbl[])
      n58 = call "PicoScopeAdcToVolts.vi"("Max_adc"=w163, "Range Index"=w152, "Data"=w153) -> ("Data"=w137:dbl[])
      n59 = call "ReadBuffer.vi"("Pointer and BufferSize"=w100, "Buffer size"=w102, "error in (no error)"=w105) -> ("Output Array"=→"overflow":i16[], "error out"=w104:errorcluster)  [unwired: 11 in]
      n60 = Bundle(0, w114, "Data"=w116) -> (w155:cluster{i32, dbl, "Data":dbl[]})  [unwired: 1 in]
      n61 = Bundle(0, w114, "Data"=w156) -> (w154:cluster{i32, dbl, "Data":dbl[]})  [unwired: 1 in]
      n62 = Bundle(0, w114, "Data"=w137) -> (w130:cluster{i32, dbl, "Data":dbl[]})  [unwired: 1 in]
      n63 = Bundle(0, w114, "Data"=w135) -> (w128:cluster{i32, dbl, "Data":dbl[]})  [unwired: 1 in]
      n64 = Bundle(0, w114, "Data"=w131) -> (w127:cluster{i32, dbl, "Data":dbl[]})  [unwired: 1 in]
      n65 = Bundle(0, w114, "Data"=w132) -> (w126:cluster{i32, dbl, "Data":dbl[]})  [unwired: 1 in]
      n66 = Bundle(0, w114, "Data"=w136) -> (w129:cluster{i32, dbl, "Data":dbl[]})  [unwired: 1 in]
      n67 = Bundle(0, w114, "Data"=w138) -> (w125:cluster{i32, dbl, "Data":dbl[]})  [unwired: 1 in]
      n68 = call-poly <vilib>:"Analog to Digital.vi"("data format (offset binary)"=w123, "full-scale range (pk-pk)"=256.0, "resolution (16 bit)"=8, "analog waveform"=w120) -> ("digital waveform"=w117:digitalwaveform)  [unwired: 4 in, 3 out]
      n69 = Or(x="Stop Display", y="Run") -> (x .or. y?=w108:bool)
      n70 = local write "Capture Complete"(TRUE ("Capture Complete")) -> ()
      n71 = Build Array(w155, w154, w130, w129, w128, w127, w126, w125) -> (w98:cluster{i32, dbl, "Data":dbl[]}[])
      "Analog Channels" <- w98
      n72 = Bundle By Name("t0"=timestamp(0 s since 1904-01-01), "dt"=w114, "Y"=w117) -> (→"Port 0":digitalwaveform)  [unwired: 1 in]
      n73 = Wait (ms)(milliseconds to wait=u32 100) -> ()  [unwired: 1 out]
    }
    n74 = case shown="True" "Write to file" {
      tunnel: w33 -> [w91 w97]
      tunnel: w32 -> [w92 w96]
      tunnel: w30 -> [_ w95]
      tunnel: [w91 w94] -> w29
      tunnel: [w92 w93] -> w28
      frame False {
      }
      frame True {
        n75 = call "PicoWriteTDMS.vi"("error in (no error)"=w96, "Analog Channels"=w95, "Refnum in"=w97) -> ("error out"=w93:errorcluster, "Refnum out"=w94:refnum<k34>)  [unwired: 7 in]
      }
    }
    n76 = call "ReleaseBuffer.vi"("error in (no error)"=w28, "Pointer and BufferSize"=w46) -> ("error out"=w45:errorcluster)  [unwired: 9 in]
    "Capture Complete" <- FALSE ("Capture Complete")
  }
  n77 = TDMS Close(11:w6) -> ()  [unwired: 1 in, 2 out]
  n78 = call "PicoScopeospaClose.vi"("error in (no error)"=w15, "handle in"=w14) -> ("error out"=w13:errorcluster)  [unwired: 8 in, 1 out]
  n79 = call "PicoReleaseMultiBuffers.vi"("error in (no error)"=w13, "Enabled array"=w16, "Data Pointers"=w1) -> ("error out"=→"error out":errorcluster)  [unwired: 7 in, 1 out]
